vi "LT_set_param.vi"(5 "PWE_in":i32, 6 "param_index":u16 step=1, 7 "param_number":u16=1 min=1 step=1, 8 "error in":errorcluster, 9 "check_readback":bool, 10 "dev_param_in":T1={"Length of data block (14)"=14, "Converter address (0)"=0, "Converter type\n(180: Turbovac 350/450 i)"=180, "PZD1 STW, ZSW (0)"=0, "PZD2 HSW, HIW (0)"=0} {"Converter type\n(180: Turbovac 350/450 i)" items=["Turbovac 350/450 i"=180, "Turbovac 350/450 i with optional interface"=181, "Turbovac 350/450 iX"=182, "Turbovac  90/250 i"=190, "Turbovac  90/250 with optional interface"=191, "Turbovac  90/250 iX"=192, "Turbovac  850/950 i"=195, "Turbovac  850/950 i with optional interface"=196, "Turbovac  850/950 iX"=197, "Turbovac 1350/1450 i"=185, "Turbovac 1350/1450 i with optional interface"=186, "Turbovac 1350/1450 iX"=187]; "Length of data block (14)" items=["14"=14, "22"=22]}, 11 "VISA in":refnum<visa-resource-name>="COM43") -> (0 "error out":errorcluster, 2 "dev_param_out":T3={"Length of data block"=14, "Converter address"=0, "Converter type"=180, "PZD1"=0, "PZD2"=0} {"Converter type" items=["Turbovac 350/450 i"=180, "Turbovac 350/450 i with optional interface"=181, "Turbovac 350/450 iX"=182, "Turbovac  90/250 i"=190, "Turbovac  90/250 with optional interface"=191, "Turbovac  90/250 iX"=192, "Turbovac  850/950 i"=195, "Turbovac  850/950 i with optional interface"=196, "Turbovac  850/950 iX"=197, "Turbovac 1350/1450 i"=185, "Turbovac 1350/1450 i with optional interface"=186, "Turbovac 1350/1450 iX"=187]; "Length of data block" items=["14"=14, "22"=22]}, 3 "VISA out":refnum<visa-resource-name>, 4 "status":bool)   [LabVIEW 2019]
doc: "Example VI to demonstrate the use of the Oerlikon Leybold TMP driver."
uses:
  <instrlib>/Leybold TURBOVAC/Public/Ctl/Device Parameters Indicator.ctl
  <instrlib>/Leybold TURBOVAC/Public/Ctl/Converter Type Indicator.ctl
  <instrlib>/Leybold TURBOVAC/Public/Ctl/Device Parameters Control.ctl
  <instrlib>/Leybold TURBOVAC/Public/Ctl/Converter Type Control.ctl
  <instrlib>/Leybold TURBOVAC/Leybold TURBOVAC.lvlib
panel:
  in  "Type of parameter access (2)":u8(ring)=2 items=["Do nothing"=0, "Parameter value"=1, "Write 16 bit value"=2, "Write 32 bit value"=3, "Field value requested"=6, "Write 16 bit field value"=7, "Write 32 bit field value"=8, "Request No. of field elements"=9]
  out "PWE out":i32
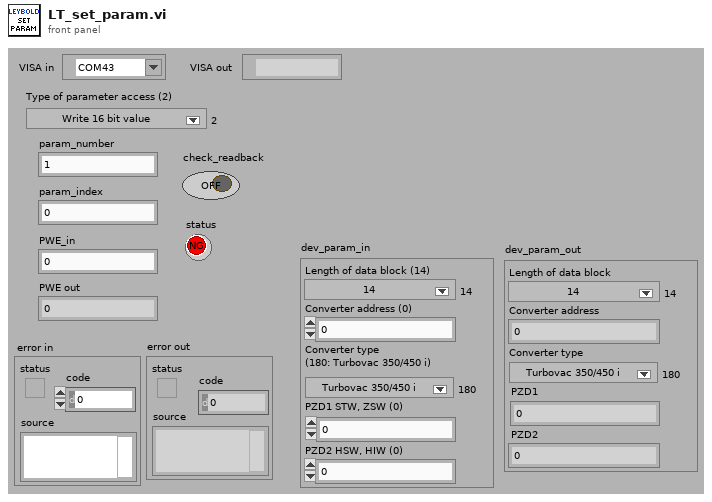
[diagram p1: front panel]
types:
  T1 = typedef "Leybold TURBOVAC.lvlib/Device Parameters Control.ctl" = cluster{"Length of data block (14)":u8, "Converter address (0)":u8, "Converter type\n(180: Turbovac 350/450 i)":T2, "PZD1 STW, ZSW (0)":u16, "PZD2 HSW, HIW (0)":u16}
  T2 = typedef "Leybold TURBOVAC.lvlib/Converter Type Control.ctl" = u16
  T3 = typedef "Leybold TURBOVAC.lvlib/Device Parameters Indicator.ctl" = cluster{"Length of data block":u8, "Converter address":u8, "Converter type":T4, "PZD1":u16, "PZD2":u16}
  T4 = typedef "Leybold TURBOVAC.lvlib/Converter Type Indicator.ctl" = u16
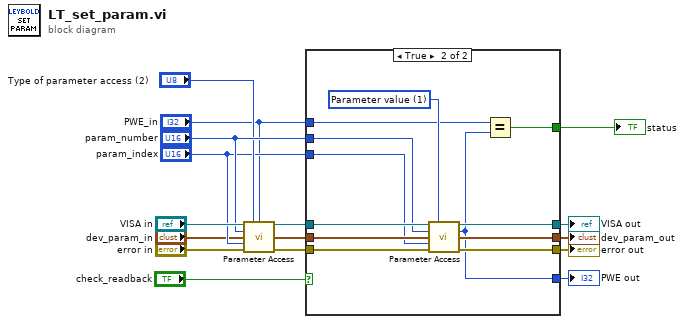
[diagram p0: block diagram]
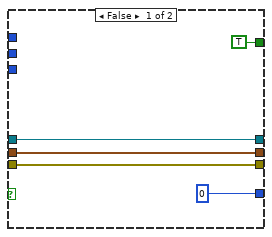
[diagram p2: hidden frame]
diagram:
  n1 = call <instrlib>:"Parameter Access.vi"("VISA resource name"="VISA in", "Type of parameter access (1: Parameter value)"="Type of parameter access (2)", "PWE (0)"="PWE_in", "PKE-PM No. (1)"="param_number", "Device parameters"="dev_param_in", "Index (0)"="param_index", "error in (no error)"="error in") -> ("VISA resource name out"=w13:refnum<visa-resource-name>, "Device parameters out"=w15:T3, "error out"=w14:errorcluster)  [unwired: 5 in, 1 out]
  n2 = case shown="True" "check_readback" {
    tunnel: w15 -> [w20 w33]
    tunnel: w14 -> [w19 w32]
    tunnel: w13 -> [w21 w31]
    tunnel: "param_number" -> [_ w29]
    tunnel: [0 ("PWE out") w23] -> w11
    tunnel: "param_index" -> [_ w28]
    tunnel: [w21 w27] -> w8
    tunnel: [w20 w26] -> w7
    tunnel: [w19 w25] -> w6
    tunnel: "PWE_in" -> [_ w24]
    tunnel: [TRUE w22] -> w1
    frame False {
    }
    frame True {
      w30 = u8 1 items=["Do nothing"=0, "Parameter value"=1, "Write 16 bit value"=2, "Write 32 bit value"=3, "Field value requested"=6, "Write 16 bit field value"=7, "Write 32 bit field value"=8, "Request No. of field elements"=9] ("Type of parameter access (1: Parameter value)")
      n3 = call <instrlib>:"Parameter Access.vi"("VISA resource name"=w31, "Type of parameter access (1: Parameter value)"=w30, "PKE-PM No. (1)"=w29, "Device parameters"=w33, "Index (0)"=w28, "error in (no error)"=w32) -> ("VISA resource name out"=w27:refnum<visa-resource-name>, "PWE out"=w23:i32, "Device parameters out"=w26:T3, "error out"=w25:errorcluster)  [unwired: 6 in]
      n4 = Equal?(x=w24, y=w23) -> (x = y?=w22:bool)
    }
  }
  "PWE out" <- w11
  "VISA out" <- w8
  "dev_param_out" <- w7
  "error out" <- w6
  "status" <- w1
